vi "Add Trigger for Acyclic Frame.vi"(8 "error in":errorcluster, 10 "acyclic frame names":string[](array[string]), 11 "bus controller in":T1 format="%.0x") -> (0 "error out":errorcluster, 3 "bus controller out":T1 format="%.0x")   [LabVIEW 2020, in "Ballard MIL-STD-1553 Scripting.lvlib"]
uses:
  Ballard MIL-STD-1553 Scripting.lvlib
  <vilib>/NI VeriStand/Custom Device API/Custom Device Item Ref.ctl
  Constants.vi
  <vilib>/NI VeriStand/Custom Device API/Custom Device API.lvlib
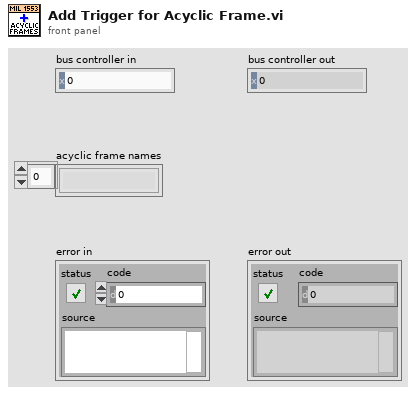
[diagram p1: front panel]
types:
  T1 = typedef "Custom Device API.lvlib/Custom Device Item Ref.ctl" = u64
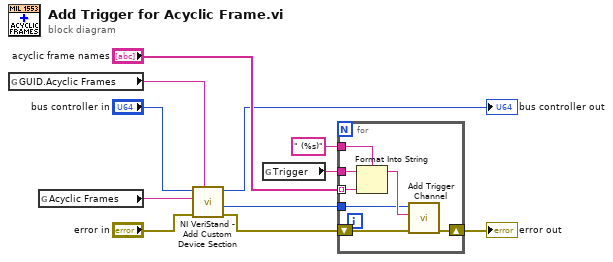
[diagram p0: block diagram]
diagram:
  n1 = global read "Constants.vi" "GUID.Acyclic Frames"() -> (w5:string)
  n2 = global read "Constants.vi" "Acyclic Frames"() -> (w4:string)
  n3 = call <vilib>:"NI VeriStand - Add Custom Device Section.vi"("GUID (Default Section)"=w5, "error in (no error)"="error in", "Section Name"=w4, "Parent Ref in"="bus controller in") -> ("error out"=w2:errorcluster, "Section Ptr"=w1:T1, "Parent Ref out"=→"bus controller out":T1)  [unwired: 4 in, 1 out]
  n4 = global read "Constants.vi" "Trigger"() -> (w11:string)
  n5 = for {
    tunnel: w11 -> [w18]
    tunnel: " (%s)" ("format string") -> [w17]
    shift-right: [w14] -> w9
    shift-left: w2 -> [w15]
    tunnel: "acyclic frame names" -> [w13] mode=indexing
    tunnel: w1 -> [w12]
    n6 = Format Into String(format string=w17, initial string=w18, w13) -> (resulting string=w16:string)  [unwired: 1 in, 1 out]
    n7 = call "Add Trigger Channel.vi"("error in"=w15, "name"=w16, "acyclic frames section in"=w12) -> ("error out"=w14:errorcluster)  [unwired: 7 in, 1 out]
  }
  "error out" <- w9
